vi "Source A.vi"() -> ()   [LabVIEW 2016]
doc: "This vi allows the user to control the beamline elements on the high voltage deck. It uses the GRoup3 controllers to access all three high voltage decks. The preacc and injector image faraday cup are controlled by the low end compact rio"
uses:
  save load/SaveLoad.lvlib
  save load/saveloadprev.ctl
panel:
  in  "Tab Control":T1(tab)
  in  "Preview-Save-Load":T2
  out "Boolean":bool
  in  "Oven i":dbl
  in  "Y Steerer":dbl(slide) scale=-500.0..500.0
  in  "Pre-Acc":dbl(slide) scale=0.0..63.0
  in  "Einzel 2":dbl(slide) scale=0.0..10.0
  in  "X Steerer":dbl(slide) scale=-500.0..500.0
  in  "Einzel 1":dbl(slide) scale=0.0..12.0
  in  "Extractor":dbl(slide) scale=0.0..26.0
  in  "Immersion Lens":dbl(slide) scale=0.0..1.0
  out "Einzel 2 display":bool
  out "Cathode display":bool
  out "Oven display":bool
  out "Einzel 1 display":bool
  out "Immersion lens display":bool
  out "Steerer display":bool
  out "Pre acc display":bool=TRUE
  in  "Cathode V":dbl(slide) scale=0.0..12.0
  out "Cathode  cluster":T3 {"Cathode" format="%#_3g"; "Cathode\nVoltage" format="%#.2g"; "Cathode \nCurrent" format="%#.2g"}
  out "Extractor  cluster":T4 {"Extractor" format="%#_3g"; "Extractor \nVoltage" format="%#.2g"; "Extractor\n Current" format="%#.2g"}
  out "Immersion Lens  cluster":T5 {"Immersion Lens" format="%#_3g"; "Immersion Lens\nCurrent" format="%#.2g"; "Immersion Lens\nVoltage" format="%#.2g"}
  in  "stop":bool
  out "Oven cluster":T6 {"Oven V" format="%#.2g"; "Oven power" format="%#.2g"; "Oven  I readback" format="%#.2g"; "Oven Current\n Set point" format="%#.2g"}
  out "Einzel 1  cluster":T7 {"Einzel 1 Voltage" format="%#.2g"; "Einzel  Current" format="%#.2g"}
  out "Source Steerer cluster":T8 {"X steerer" format="%#.2g"; "Y Steerer" format="%#.2g"}
  out "Einzel 2  cluster":T9 {"Einzel 2 voltage" format="%#.2g"; "Einzel 2 Current" format="%#.2g"}
  out "Preacc cluster":T10 {"Pre-acc Voltage" format="%#.2g"; "Pre-acc current" format="%#.2g"}
  out "Cryo pump":T11
  out "Ion gauge Cluster 1":T12
  out "sample change finished change":bool
  out "chop voltage":dbl
  in  "reset oven":bool
  out "Extractor display":bool
  out "pre-acc set":dbl format="%#_3g"
  out "Pre-acc Voltage":dbl format="%#_3g"
  out "Pre-acc current":dbl format="%#_3g"
  out "inj cup out":bool
  out "Output Current":dbl format="%.4f"
  out "Output Power":dbl format="%.4f"
  out "Output Voltage":dbl format="%.4f"
  out "Read Set Current":dbl format="%.4f"
  out "Read Set Voltage":dbl format="%.4f"
  out "ID responce":string
  out "Address \"OK\"":string
  in  "Source A temp file":path=path "D:/Main Tune Parameters/Temp Configs/Source A.txt"
  out "Oven readback error":errorcluster
  out "SaveLoad error":errorcluster
  out "Oven Reset Error":errorcluster
  out "Oven Set Error":errorcluster
  out "SV error":errorcluster
  # "Source A"
  # "red is in the beamline\nblue is out of the beamline"
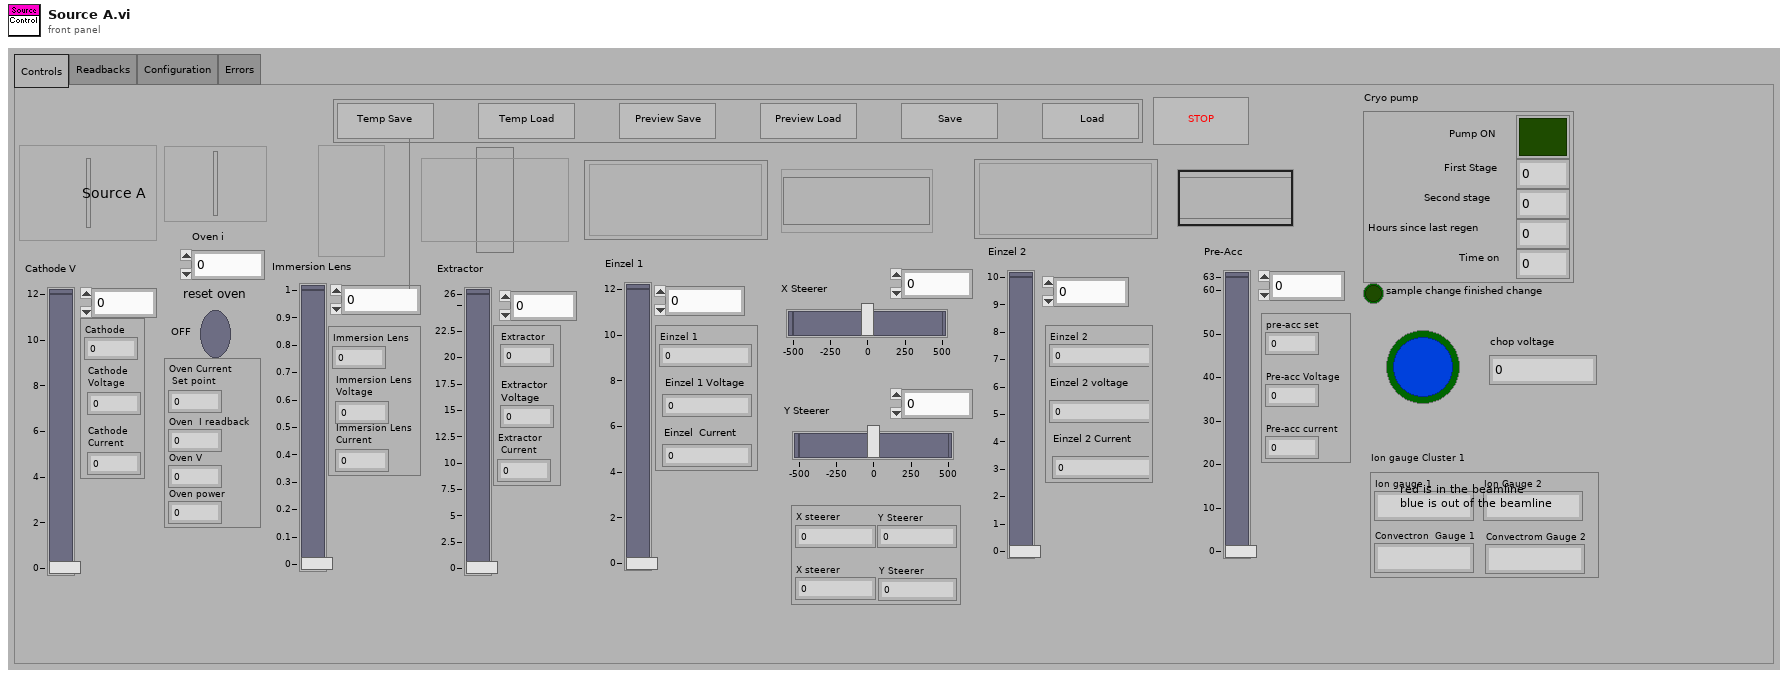
[diagram p1: front panel]
types:
  T1 = enum32{"Controls", "Readbacks", "Configuration", "Errors"}
  T2 = typedef "saveloadprev.ctl" = cluster{"Temp Save":bool, "Temp Load":bool, "Save":bool, "Load":bool, "Preview Save":bool, "Preview Load":bool}
  T3 = cluster{"Cathode":dbl, "Cathode\nVoltage":dbl, "Cathode \nCurrent":dbl}
  T4 = cluster{"Extractor":dbl, "Extractor \nVoltage":dbl, "Extractor\n Current":dbl}
  T5 = cluster{"Immersion Lens":dbl, "Immersion Lens\nCurrent":dbl, "Immersion Lens\nVoltage":dbl}
  T6 = cluster{"Oven  I readback":dbl, "Oven Current\n Set point":dbl, "Oven power":dbl, "Oven V ":dbl}
  T7 = cluster{"Einzel 1":dbl, "Einzel 1 Voltage":dbl, "Einzel  Current":dbl}
  T8 = cluster{"X steerer":dbl, "X steerer":dbl, "Y Steerer":dbl, "Y Steerer ":dbl}
  T9 = cluster{"Einzel 2":dbl, "Einzel 2 voltage":dbl, "Einzel 2 Current":dbl}
  T10 = cluster{"pre-acc set":dbl, "Pre-acc Voltage":dbl, "Pre-acc current":dbl}
  T11 = cluster{"First Stage":dbl, "Second stage":dbl, "Hours since last regen":dbl, "Pump ON":bool, "Time on":dbl}
  T12 = cluster{"Ion gauge 1":string, "Convectron  Gauge 1 ":string, "Ion Gauge 2":string, "Convectrom Gauge 2":string}
  T13 = cluster{"X steerer":dbl, "X steerer":dbl, "Y Steerer":dbl, "Y Steerer":dbl}
  T14 = cluster{"Einzel 1":dbl, "Einzel 1\nVoltage":dbl, "Einzel \nCurrent":dbl}
  T15 = cluster{"Pre-Acc":dbl, "Double":dbl, "Double":dbl}
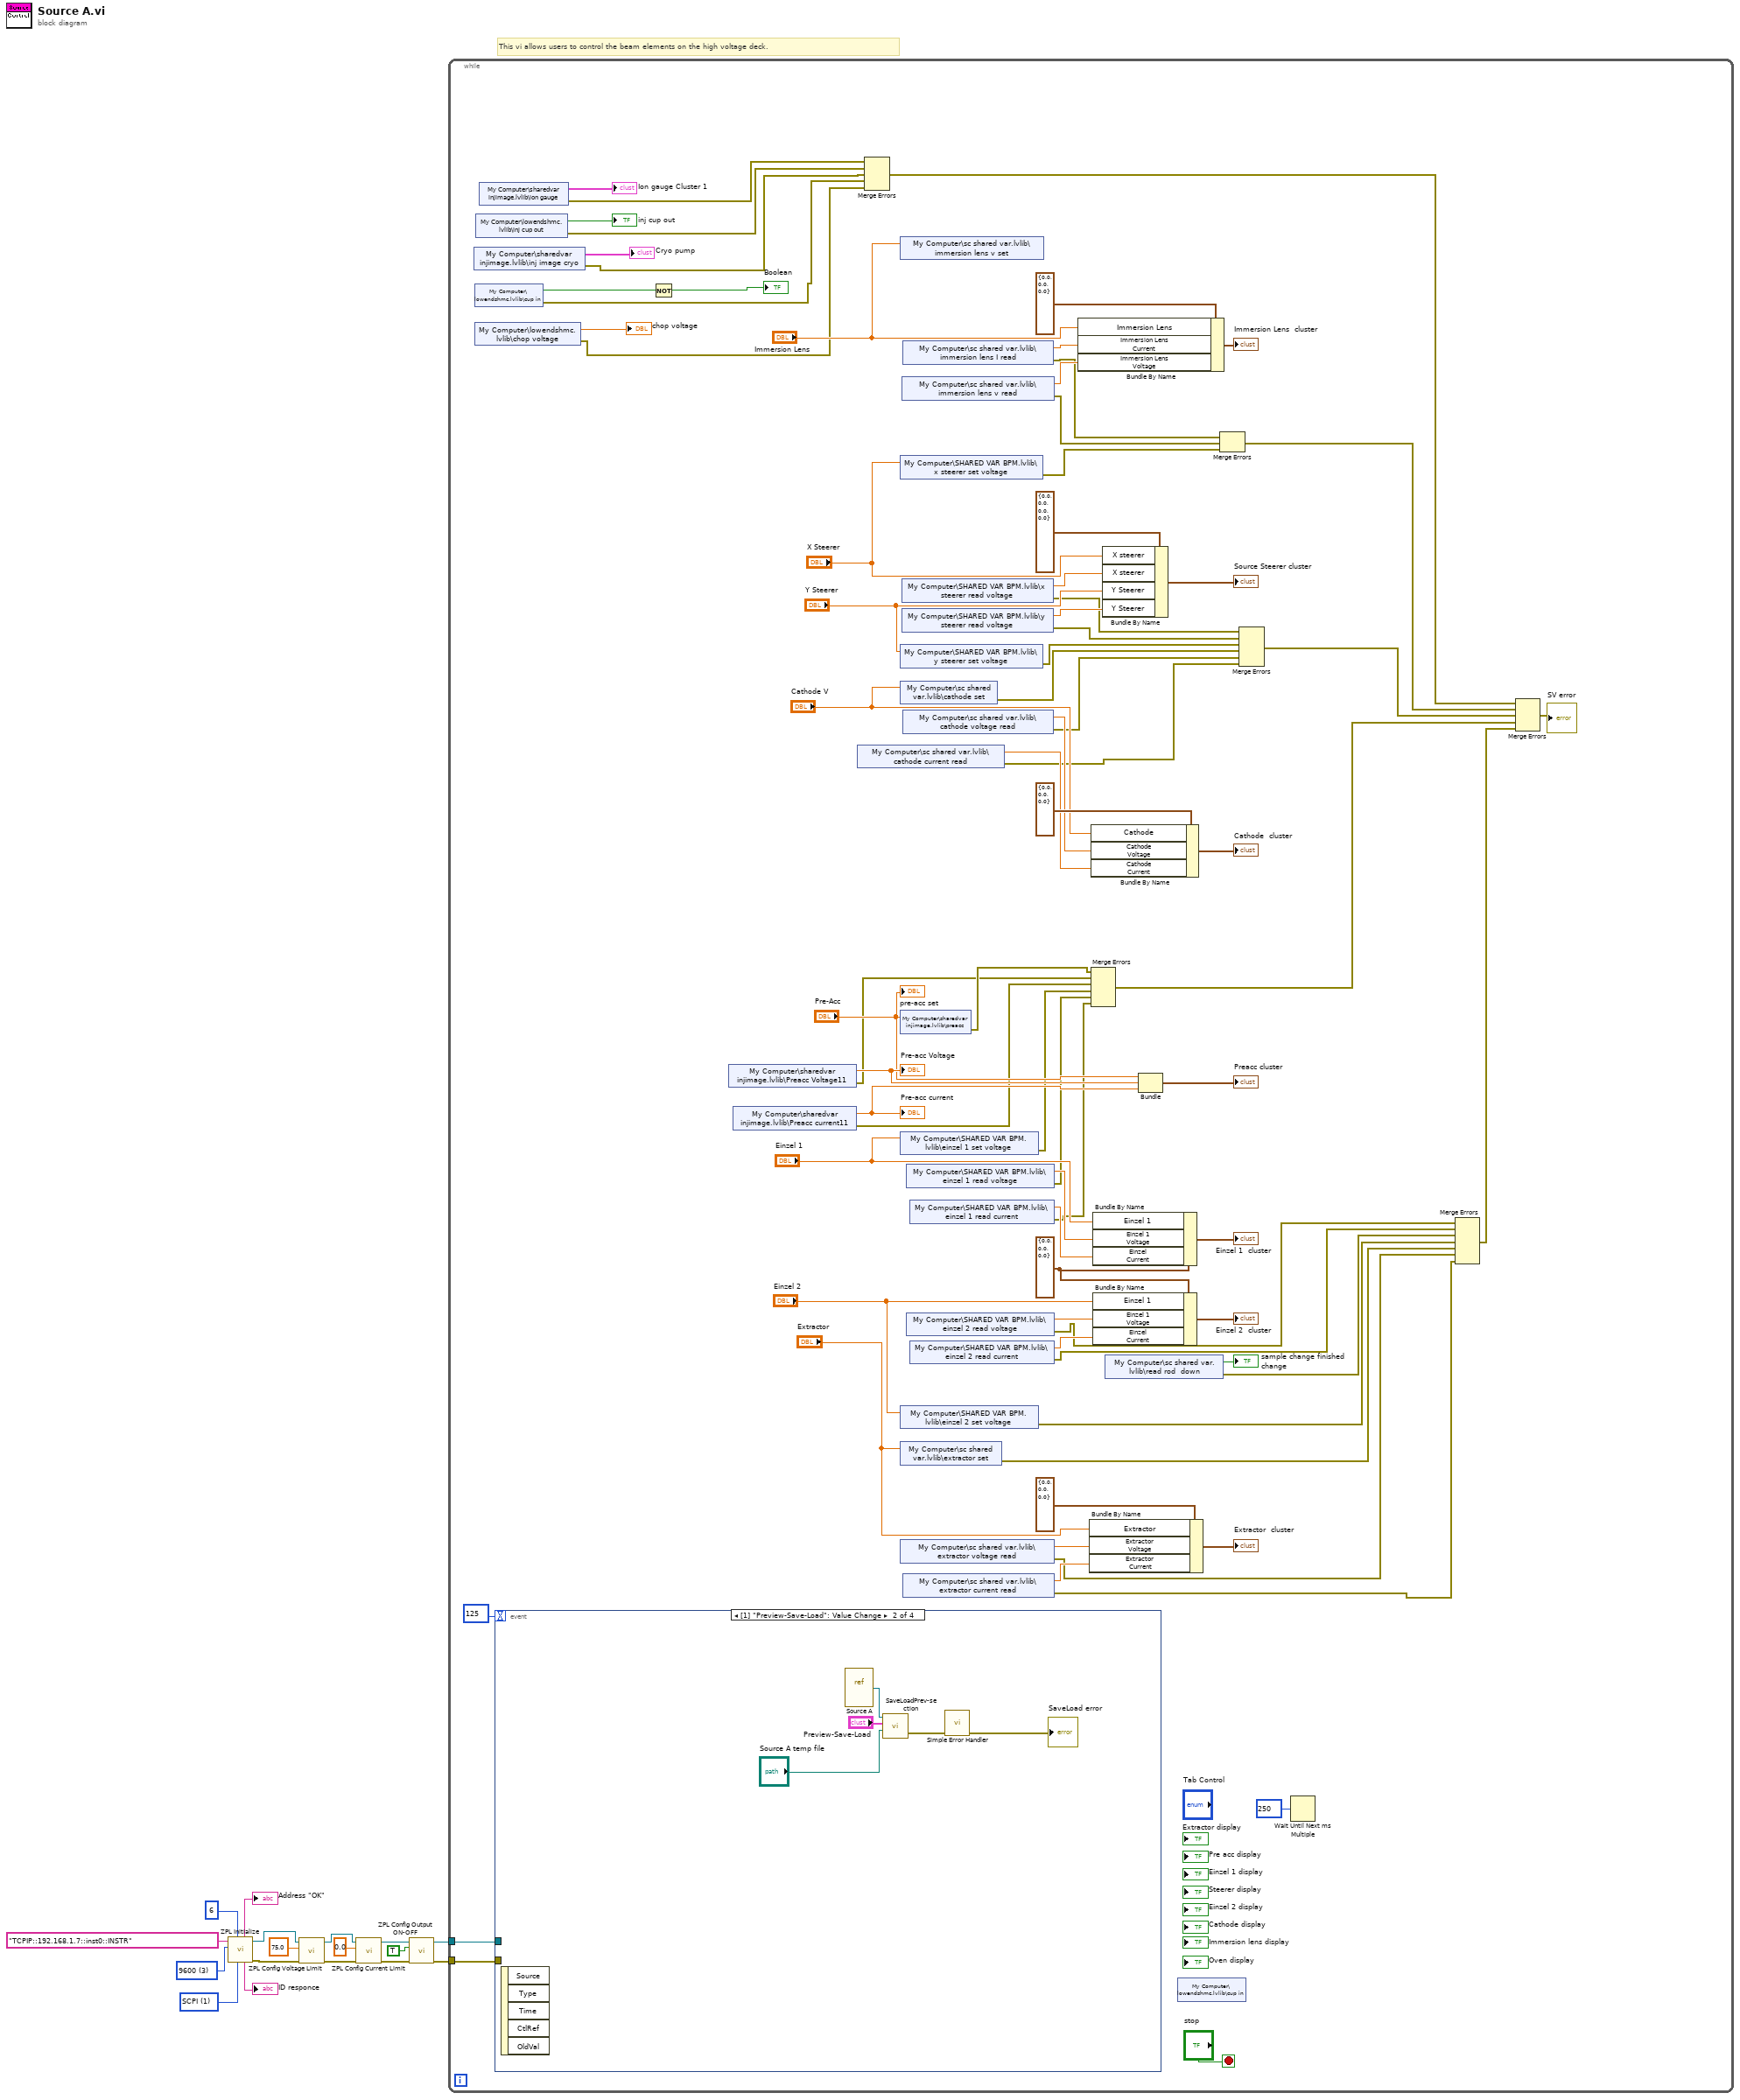
[diagram p0: block diagram]
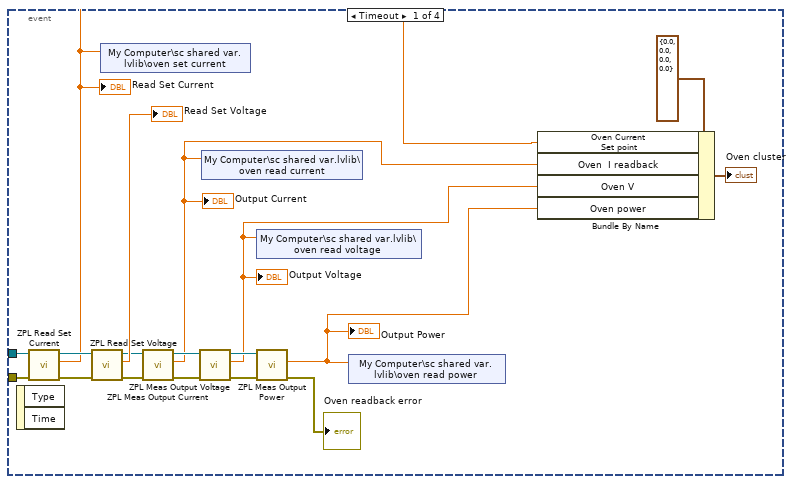
[diagram p2: hidden frame]
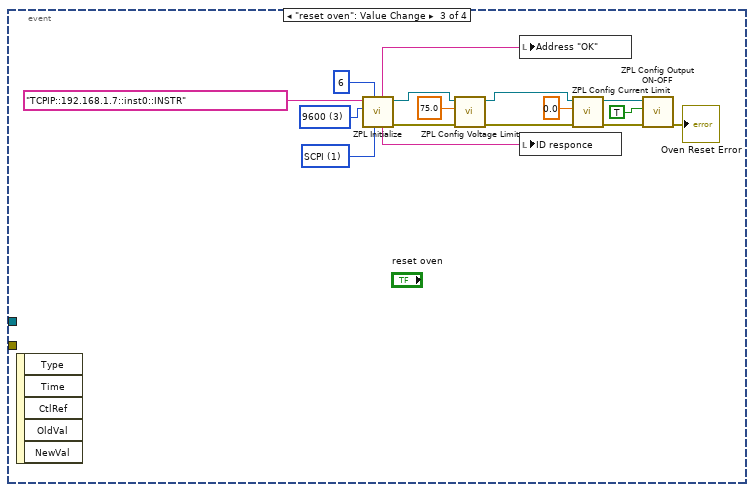
[diagram p3: hidden frame]
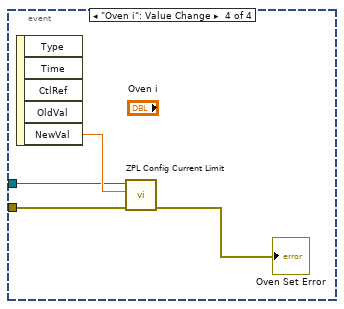
[diagram p4: hidden frame]
diagram:
  w17 = 3 items=["1200", "2400", "4800", "9600", "19200", "38400", "57600", "115200"] ("Baud Rate")
  w16 = i16 1 items=["GEN", "SCPI"] ("Language Selector")
  # "This vi allows users to control the beam elements on the high voltage deck."
  n1 = call "ZPL Initialize.vi"("Language Selector"=w16, "Address"=i16 6, "Baud Rate"=w17, "VISA"="TCPIP::192.168.1.7::inst0::INSTR" ("format string")) -> ("error out"=w7:errorcluster, "VISA  out"=w8:refnum<visa-resource-name>, "ID responce"=→"ID responce":string, "Address \"OK\""=→"Address \"OK\"":string)  [unwired: 4 in]
  n2 = call "ZPL Config Voltage Limit.vi"("error"=w7, "Voltage Limit"=75.0, "VISA"=w8) -> ("error out"=w9:errorcluster, "VISA out"=w10:refnum<visa-resource-name>)  [unwired: 7 in]
  n3 = call "ZPL Config Current Limit.vi"("error"=w9, "Current Limit"=0.0, "VISA"=w10) -> ("error out"=w13:errorcluster, "VISA out"=w12:refnum<visa-resource-name>)  [unwired: 7 in]
  n4 = call "ZPL Config Output ON-OFF.vi"("error"=w13, "Output ON"=TRUE, "VISA"=w12) -> ("error out"=w4:errorcluster, "VISA out"=w5:refnum<visa-resource-name>)  [unwired: 7 in]
  n5 = while {
    tunnel: w5 -> [w75]
    tunnel: w4 -> [w74]
    stop <- "stop" stop-if-true
    w69 = T14 {"Einzel 1"=0.0, "Einzel 1\nVoltage"=0.0, "Einzel \nCurrent"=0.0} ("Einzel 1  cluster 2")
    n6 = shared-variable "My Computer\\sharedvar injimage.lvlib\\inj image cryo"() -> (→"Cryo pump":T11, error out=w48:errorcluster)  [unwired: 1 in]
    n7 = shared-variable "My Computer\\lowendshmc.lvlib\\cup in"() -> (w90:bool, error out=w47:errorcluster)  [unwired: 1 in]
    n8 = shared-variable "My Computer\\lowendshmc.lvlib\\chop voltage"() -> (→"chop voltage":dbl, error out=w46:errorcluster)  [unwired: 1 in]
    n9 = shared-variable "My Computer\\lowendshmc.lvlib\\inj cup out"() -> (→"inj cup out":bool, error out=w49:errorcluster)  [unwired: 1 in]
    n10 = shared-variable "My Computer\\sharedvar injimage.lvlib\\ion gauge"() -> (→"Ion gauge Cluster 1":cluster{string, string, string, string}, error out=w50:errorcluster)  [unwired: 1 in]
    n11 = event shown="[1] \"Preview-Save-Load\": Value Change" {
      selector: _ -> [_ _ _ _]
      dyn-events: _ -> [_ _ _ _]
      timeout: 125 -> [_ _ _ _]
      tunnel: w75 -> [w104 _ _ w137]
      tunnel: w74 -> [w103 _ _ w138]
      event Timeout {
        n12 = event-data() -> ()  [unwired: 1 in, 2 out]
        n13 = call "ZPL Read Set Current.vi"("error"=w103, "VISA"=w104) -> ("error out"=w114:errorcluster, "Read Set Current"=w99:dbl, "VISA out"=w113:refnum<visa-resource-name>)  [unwired: 7 in]
        "Read Set Current" <- w99
        n14 = call "ZPL Read Set Voltage.vi"("error"=w114, "VISA"=w113) -> ("error out"=w110:errorcluster, "Read Set Voltage"=→"Read Set Voltage":dbl, "VISA out"=w111:refnum<visa-resource-name>)  [unwired: 7 in]
        n15 = shared-variable "My Computer\\sc shared var.lvlib\\oven set current"(w99) -> ()  [unwired: 1 in, 1 out]
        n16 = call "ZPL Meas Output Current.vi"("error"=w110, "VISA"=w111) -> ("error out"=w108:errorcluster, "Output Current"=w100:dbl, "VISA out"=w109:refnum<visa-resource-name>)  [unwired: 7 in]
        "Output Current" <- w100
        n17 = call "ZPL Meas Output Voltage.vi"("error"=w108, "VISA"=w109) -> ("error out"=w106:errorcluster, "Output Voltage"=w98:dbl, "VISA out"=w107:refnum<visa-resource-name>)  [unwired: 7 in]
        "Output Voltage" <- w98
        n18 = shared-variable "My Computer\\sc shared var.lvlib\\oven read current"(w100) -> ()  [unwired: 1 in, 1 out]
        n19 = shared-variable "My Computer\\sc shared var.lvlib\\oven read voltage"(w98) -> ()  [unwired: 1 in, 1 out]
        n20 = call "ZPL Meas Output Power.vi"("error"=w106, "VISA"=w107) -> ("error out"=→"Oven readback error":errorcluster, "Output Power"=w97:dbl)  [unwired: 7 in, 1 out]
        "Output Power" <- w97
        n21 = shared-variable "My Computer\\sc shared var.lvlib\\oven read power"(w97) -> ()  [unwired: 1 in, 1 out]
        n22 = Bundle By Name(cluster=T6 {"Oven  I readback"=0.0, "Oven Current\n Set point"=0.0, "Oven power"=0.0, "Oven V "=0.0} ("Oven cluster"), "Oven Current\n Set point"=w99, "Oven  I readback"=w100, "Oven V"=w98, "Oven power"=w97) -> (→"Oven cluster":T6)
      }
      event Value Change {
        n23 = event-data() -> ()  [unwired: 1 in, 5 out]
        n24 = vi-ref "Source A.vi"() -> (w117:refnum<vi>)
        n25 = call "SaveLoadPrev-section.vi"("file path (use dialog)"="Source A temp file", "Cluster 2"="Preview-Save-Load", "VI Refnum"=w117) -> ("error out"=w116:errorcluster)  [unwired: 2 in]
        n26 = call <vilib>:"Simple Error Handler.vi"("error in (no error)"=w116) -> ("error out"=→"SaveLoad error":errorcluster)  [unwired: 4 in, 4 out]
      }
      event "reset oven": Value Change {
        w124 = 3 items=["1200", "2400", "4800", "9600", "19200", "38400", "57600", "115200"] ("Baud Rate")
        w125 = i16 1 items=["GEN", "SCPI"] ("Language Selector")
        n27 = event-data() -> ()  [unwired: 1 in, 5 out]
        n28 = call "ZPL Initialize.vi"("Language Selector"=w125, "Address"=i16 6, "Baud Rate"=w124, "VISA"="TCPIP::192.168.1.7::inst0::INSTR" ("format string")) -> ("error out"=w133:errorcluster, "VISA  out"=w132:refnum<visa-resource-name>, "ID responce"=w121:string, "Address \"OK\""=w122:string)  [unwired: 4 in]
        n29 = call "ZPL Config Voltage Limit.vi"("error"=w133, "Voltage Limit"=75.0, "VISA"=w132) -> ("error out"=w131:errorcluster, "VISA out"=w130:refnum<visa-resource-name>)  [unwired: 7 in]
        n30 = local write "Address \"OK\""(w122) -> ()
        n31 = local write "ID responce"(w121) -> ()
        n32 = call "ZPL Config Current Limit.vi"("error"=w131, "Current Limit"=0.0, "VISA"=w130) -> ("error out"=w127:errorcluster, "VISA out"=w128:refnum<visa-resource-name>)  [unwired: 7 in]
        n33 = call "ZPL Config Output ON-OFF.vi"("error"=w127, "Output ON"=TRUE, "VISA"=w128) -> ("error out"=→"Oven Reset Error":errorcluster)  [unwired: 7 in, 1 out]
      }
      event "Oven i": Value Change {
        n34 = event-data() -> ("NewVal"=w139:dbl)  [unwired: 1 in, 4 out]
        n35 = call "ZPL Config Current Limit.vi"("error"=w138, "Current Limit"=w139, "VISA"=w137) -> ("error out"=→"Oven Set Error":errorcluster)  [unwired: 7 in, 1 out]
      }
    }
    n36 = Not(x=w90) -> (.not. x?=→"Boolean":bool)
    n37 = shared-variable "My Computer\\sharedvar injimage.lvlib\\Preacc Voltage11"() -> (w55:dbl, error out=w32:errorcluster)  [unwired: 1 in]
    "Pre-acc Voltage" <- w55
    n38 = shared-variable "My Computer\\sharedvar injimage.lvlib\\Preacc current11"() -> (w53:dbl, error out=w31:errorcluster)  [unwired: 1 in]
    "Pre-acc current" <- w53
    n39 = shared-variable "My Computer\\sc shared var.lvlib\\cathode current read"() -> (w77:dbl, error out=w37:errorcluster)  [unwired: 1 in]
    n40 = Merge Errors(w50, w49, w48, w47, w46) -> (w36:errorcluster)
    n41 = shared-variable "My Computer\\sc shared var.lvlib\\immersion lens v set"("Immersion Lens") -> ()  [unwired: 1 in, 1 out]
    n42 = shared-variable "My Computer\\SHARED VAR BPM.lvlib\\x steerer set voltage"("X Steerer") -> (error out=w43:errorcluster)  [unwired: 1 in]
    n43 = shared-variable "My Computer\\SHARED VAR BPM.lvlib\\y steerer set voltage"("Y Steerer") -> (error out=w40:errorcluster)  [unwired: 1 in]
    n44 = shared-variable "My Computer\\sc shared var.lvlib\\cathode set"("Cathode V") -> (error out=w39:errorcluster)  [unwired: 1 in]
    n45 = shared-variable "My Computer\\sharedvar injimage.lvlib\\preacc"("Pre-Acc") -> (error out=w33:errorcluster)  [unwired: 1 in]
    n46 = shared-variable "My Computer\\SHARED VAR BPM.lvlib\\einzel 1 set voltage"("Einzel 1") -> (error out=w30:errorcluster)  [unwired: 1 in]
    n47 = shared-variable "My Computer\\SHARED VAR BPM.lvlib\\einzel 2 set voltage"("Einzel 2") -> (error out=w23:errorcluster)  [unwired: 1 in]
    n48 = shared-variable "My Computer\\sc shared var.lvlib\\extractor set"("Extractor") -> (error out=w22:errorcluster)  [unwired: 1 in]
    n49 = shared-variable "My Computer\\sc shared var.lvlib\\extractor voltage read"() -> (w83:dbl, error out=w21:errorcluster)  [unwired: 1 in]
    n50 = shared-variable "My Computer\\sc shared var.lvlib\\immersion lens v read"() -> (w56:dbl, error out=w44:errorcluster)  [unwired: 1 in]
    n51 = shared-variable "My Computer\\SHARED VAR BPM.lvlib\\x steerer read voltage"() -> (w62:dbl, error out=w42:errorcluster)  [unwired: 1 in]
    n52 = shared-variable "My Computer\\SHARED VAR BPM.lvlib\\y steerer read voltage"() -> (w60:dbl, error out=w41:errorcluster)  [unwired: 1 in]
    n53 = shared-variable "My Computer\\sc shared var.lvlib\\immersion lens I read"() -> (w57:dbl, error out=w45:errorcluster)  [unwired: 1 in]
    n54 = shared-variable "My Computer\\sc shared var.lvlib\\cathode voltage read"() -> (w78:dbl, error out=w38:errorcluster)  [unwired: 1 in]
    n55 = shared-variable "My Computer\\sc shared var.lvlib\\extractor current read"() -> (w81:dbl, error out=w20:errorcluster)  [unwired: 1 in]
    n56 = shared-variable "My Computer\\SHARED VAR BPM.lvlib\\einzel 1 read voltage"() -> (w73:dbl, error out=w29:errorcluster)  [unwired: 1 in]
    n57 = shared-variable "My Computer\\SHARED VAR BPM.lvlib\\einzel 2 read voltage"() -> (w66:dbl, error out=w26:errorcluster)  [unwired: 1 in]
    n58 = shared-variable "My Computer\\SHARED VAR BPM.lvlib\\einzel 1 read current"() -> (w72:dbl, error out=w28:errorcluster)  [unwired: 1 in]
    n59 = shared-variable "My Computer\\SHARED VAR BPM.lvlib\\einzel 2 read current"() -> (w65:dbl, error out=w25:errorcluster)  [unwired: 1 in]
    n60 = Bundle By Name(cluster=T5 {"Immersion Lens"=0.0, "Immersion Lens\nCurrent"=0.0, "Immersion Lens\nVoltage"=0.0} ("Immersion Lens  cluster  2"), "Immersion Lens"="Immersion Lens", "Immersion Lens\nCurrent"=w57, "Immersion Lens\nVoltage"=w56) -> (→"Immersion Lens  cluster":T5)
    n61 = Bundle By Name(cluster=T4 {"Extractor"=0.0, "Extractor \nVoltage"=0.0, "Extractor\n Current"=0.0} ("Extractor  cluster"), "Extractor"="Extractor", "Extractor \nVoltage"=w83, "Extractor\n Current"=w81) -> (→"Extractor  cluster":T4)
    n62 = Bundle By Name(cluster=T3 {"Cathode"=0.0, "Cathode\nVoltage"=0.0, "Cathode \nCurrent"=0.0} ("Cathode  cluster"), "Cathode"="Cathode V", "Cathode\nVoltage"=w78, "Cathode \nCurrent"=w77) -> (→"Cathode  cluster":T3)
    n63 = Merge Errors(w33, w32, w31, w30, w29, w28) -> (w27:errorcluster)
    n64 = Bundle By Name(cluster=w69, "Einzel 1"="Einzel 1", "Einzel 1\nVoltage"=w73, "Einzel \nCurrent"=w72) -> (→"Einzel 1  cluster":T14)
    n65 = Bundle By Name(cluster=w69, "Einzel 1"="Einzel 2", "Einzel 1\nVoltage"=w66, "Einzel \nCurrent"=w65) -> (→"Einzel 2  cluster":T14)
    n66 = Bundle By Name(cluster=T13 {"X steerer"=0.0, "X steerer"=0.0, "Y Steerer"=0.0, "Y Steerer"=0.0} ("Source Steerer cluster 2"), "X steerer"="X Steerer", "X steerer"=w62, "Y Steerer"="Y Steerer", "Y Steerer"=w60) -> (→"Source Steerer cluster":T13)
    n67 = shared-variable "My Computer\\sc shared var.lvlib\\read rod  down"() -> (→"sample change finished change":bool, error out=w24:errorcluster)  [unwired: 1 in]
    n68 = Bundle("Pre-Acc"="Pre-Acc", "Double"=w55, "Double"=w53) -> (→"Preacc cluster":T15)  [unwired: 1 out]
    n69 = shared-variable "My Computer\\lowendshmc.lvlib\\cup in"() -> ()  [unwired: 1 in, 2 out]
    n70 = Merge Errors(w45, w44, w43) -> (w35:errorcluster)
    n71 = Merge Errors(w42, w41, w40, w39, w38, w37) -> (w34:errorcluster)
    n72 = Wait Until Next ms Multiple(millisecond multiple=u32 250) -> ()  [unwired: 1 out]
    n73 = Merge Errors(w26, w25, w24, w23, w22, w21, w20) -> (w19:errorcluster)
    n74 = Merge Errors(w36, w35, w34, w27, w19) -> (→"SV error":errorcluster)
    "pre-acc set" <- "Pre-Acc"
  }
